vi "PH_ForceSensor.evt Call set Ranges.vi"(0 "i ref in":refnum<vi>, 2 "Instance":string="N/A", 3 "Ranges [N]":T1, 5 "error in (no error)":errorcluster) -> (14 "i ref out":refnum<vi>, 19 "error out":errorcluster)   [LabVIEW 2014, in "PH_ForceSensor.lvlib"]
doc: "This VI sends a \"Remote Controlled Command\""
uses:
  PH_ForceSensor.lvlib
  PH_ForceSensor.Ranges.ctl
  CSCore/CSSystem/CoreLib/CoreLib.double 2 byte array.vi
  CSCore/BaseProcess/BaseProcess.lvlib
  CSCore/CSSystem/CoreLib/CoreLib.lvlib
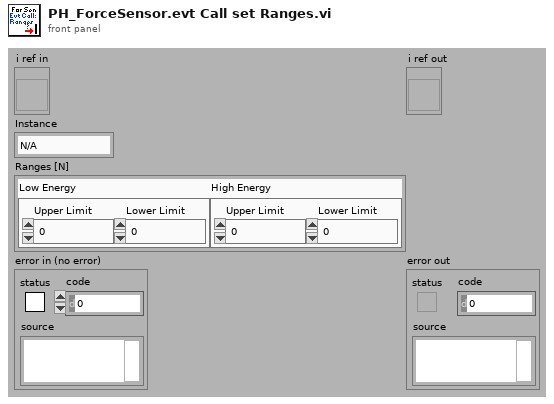
[diagram p1: front panel]
types:
  T1 = typedef "PH_ForceSensor.lvlib/PH_ForceSensor.Ranges.ctl" = cluster{"Low Energy":cluster{"Upper Limit":dbl, "Lower Limit":dbl}, "High Energy":cluster{"Upper Limit":dbl, "Lower Limit":dbl}}
  T2 = typedef "CoreDefs.rawDataType.ctl" = i8[]
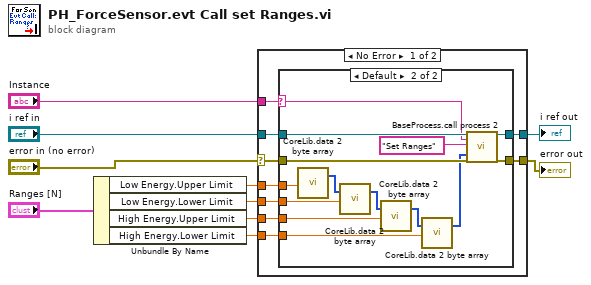
[diagram p0: block diagram]
diagram:
  n1 = Unbundle By Name("Ranges [N]") -> ("Low Energy.Upper Limit"=w4:dbl, "Low Energy.Lower Limit"=w3:dbl, "High Energy.Upper Limit"=w2:dbl, "High Energy.Lower Limit"=w1:dbl)
  n2 = case shown="No Error" "error in (no error)" {
    selector: "error in (no error)" -> [w14 w36]
    tunnel: [w19 w37] -> w10
    tunnel: [w18 w36] -> w9
    tunnel: "i ref in" -> [w17 w37]
    tunnel: w4 -> [w16 _]
    tunnel: "Instance" -> [w15 _]
    tunnel: w3 -> [w13 _]
    tunnel: w2 -> [w12 _]
    tunnel: w1 -> [w11 _]
    frame No Error {
      n3 = case shown="Default" w15 {
        selector: w15 -> [_ w30]
        tunnel: [w21 w35] -> w19
        tunnel: [w20 w34] -> w18
        tunnel: w17 -> [w21 w33]
        tunnel: w14 -> [w20 w32]
        tunnel: w16 -> [_ w29]
        tunnel: w13 -> [_ w28]
        tunnel: w12 -> [_ w27]
        tunnel: w11 -> [_ w26]
        frame "N/A" {
        }
        frame Default {
          n4 = call-poly "CoreLib.data 2 byte array.vi"("f64"=w29) -> ("byteArray out"=w25:T2)  [unwired: 18 in]
          n5 = call-poly "CoreLib.data 2 byte array.vi"("byteArray"=w25, "f64"=w28) -> ("byteArray out"=w24:T2)  [unwired: 17 in]
          n6 = call-poly "CoreLib.data 2 byte array.vi"("byteArray"=w24, "f64"=w27) -> ("byteArray out"=w23:T2)  [unwired: 17 in]
          n7 = call-poly "CoreLib.data 2 byte array.vi"("byteArray"=w23, "f64"=w26) -> ("byteArray out"=w22:T2)  [unwired: 17 in]
          n8 = call "BaseProcess.call process 2.vi"("i ref in"=w33, "Object"=w30, "Selector"="Set Ranges", "Data"=w22, "error in (no error)"=w32) -> ("i ref out"=w35:refnum<vi>, "error out"=w34:errorcluster)  [unwired: 13 in]
        }
      }
    }
    frame Error {
    }
  }
  "error out" <- w9
  "i ref out" <- w10
